vi "RSZVB Set IMOD Max Order.vi"(8 "error in (no error)":errorcluster {"code" format="%.0x"}, 9 "Max Order (3)":i32(ring)=3 items=["3"=3, "5"=5, "7"=7, "9"=9], 10 "Channel (1)":i32=1, 11 "VISA session":refnum<visa-resource-name>) -> (0 "error out":errorcluster {"code" format="%.0x"}, 3 "dup VISA session":refnum<visa-resource-name>)   [LabVIEW 2011]
doc: "This VI defines the maximum order of intermodulation products for the intermodulation spectrum measurement. \n\nNote(s):\n\n(1) This VI is not available for R&S ZVB instrument.\n\nRemote-control command(s):\n[SENSe<Ch>:]FREQuency:IMODulation:SPECtrum:MORDer"
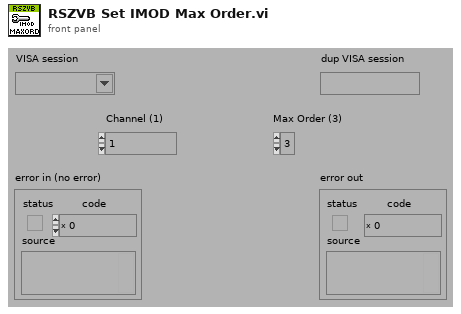
[diagram p1: front panel]
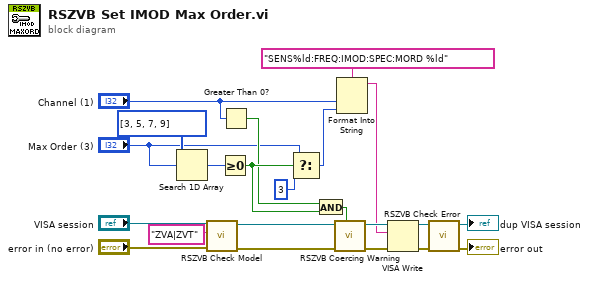
[diagram p0: block diagram]
diagram:
  n1 = Search 1D Array(1D array=i32[] [3, 5, 7, 9], element="Max Order (3)") -> (index of element=w22:i32)  [unwired: 1 in]
  n2 = call "RSZVB Check Model.vi"("error in (no error)"="error in (no error)", "Model"="ZVA|ZVT", "VISA session"="VISA session") -> ("error out"=w6:errorcluster, "dup VISA session"=w5:refnum<visa-resource-name>)  [unwired: 7 in]
  n3 = Greater Or Equal To 0?(x=w22) -> (x >= 0?=w19:bool)
  n4 = Greater Than 0?(x="Channel (1)") -> (x > 0?=w17:bool)
  n5 = Select(t="Max Order (3)", s=w19, f=3) -> (s? t:f=w21:i32)
  n6 = And(x=w17, y=w19) -> (x .and. y?=w18:bool)
  n7 = call "RSZVB Coercing Warning.vi"("In Range?"=w18, "error in (no error)"=w6, "VISA session"=w5) -> ("error out"=w13:errorcluster, "dup VISA session"=w14:refnum<visa-resource-name>)  [unwired: 7 in]
  n8 = Format Into String(format string="SENS%ld:FREQ:IMOD:SPEC:MORD %ld", "Channel (1)", w21) -> (resulting string=w12:string)  [unwired: 2 in, 1 out]
  n9 = VISA Write(VISA resource name=w14, write buffer=w12, error in (no error)=w13) -> (VISA resource name out=w11:refnum<visa-resource-name>, error out=w10:errorcluster)  [unwired: 1 out]
  n10 = call "RSZVB Check Error.vi"("error in (no error)"=w10, "VISA session"=w11) -> ("error out"=→"error out":errorcluster, "dup VISA session"=→"dup VISA session":refnum<visa-resource-name>)  [unwired: 8 in]
